vi "AlicatRestekRead.vi"(7 "Restek ProFLOW 6000 port":refnum<visa-resource-name>="ASRL3::INSTR", 11 "IP Address":string="10.245.24.172" caption="Alicat address") -> (2 "values":dbl[](array[numeric]))   [LabVIEW 2021]
panel:
  in  "AlicatRegisters":u16[](array[numeric])=[1210, 1202, 1204, 1206, 1208]
  # "MdotSP"
  # "P"
  # "T"
  # "Vol flow"
  # "mDotMeas"
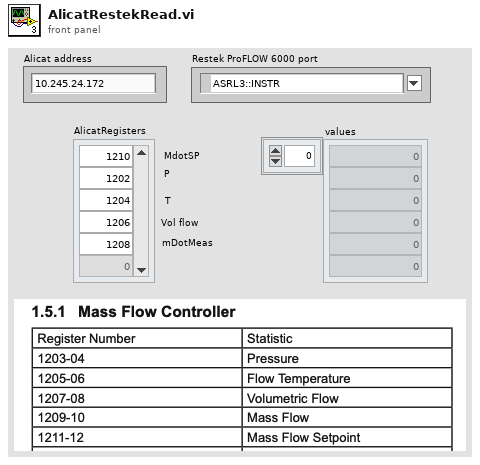
[diagram p1: front panel]
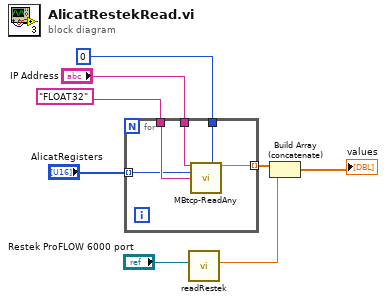
[diagram p0: block diagram]
diagram:
  n1 = for {
    tunnel: u8 0 ("Slave ID") -> [w13]
    tunnel: "FLOAT32" ("DataType(:RegisterType)") -> [w12]
    tunnel: "IP Address" -> [w11]
    tunnel: "AlicatRegisters" -> [w10] mode=indexing
    tunnel: [w9] -> w3 mode=indexing
    n2 = call "MBtcp-ReadAny.vi"("IP Address"=w11, "Slave ID"=w13, "Register"=w10, "DataType(:RegisterType)"=w12) -> ("Value"=w9:dbl)  [unwired: 9 in, 2 out]
  }
  n3 = call "readRestek.vi"("Port Name"="Restek ProFLOW 6000 port") -> ("lpm"=w1:dbl)  [unwired: 10 in]
  n4 = Build Array (concatenate)(w3, w1) -> (→"values":dbl[])
